vi "MENU_Shortcut Generate.vi"(6 "PlatMods":T3, 9 "VKey":T2, 10 "Char":i16) -> (2 "short cut":T1)   [LabVIEW 2016]
uses:
  <vilib>/event_ctls.llb/eventvkey.ctl
  <vilib>/Utility/miscctls.llb/LVMenuShortCut.ctl
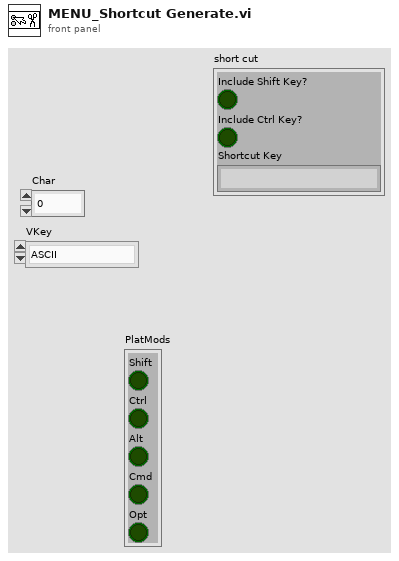
[diagram p1: front panel]
types:
  T1 = typedef "LVMenuShortCut.ctl" = cluster{"Include Shift Key?":bool, "Include Ctrl Key?":bool, "Shortcut Key":string}
  T2 = typedef "eventvkey.ctl" = enum16{"ASCII", "Enter", "Return", "Shift", "Ctrl", "Alt", "Cmd", "Opt", "Caps", "NumLock", "Clear", "Break", "Up", "Down", "Left", "Right", "Insert", "Delete", "Home", "End", "PageUp", "PageDown", "Escape", "Help", "Pause", "ScrollLock", "F1", "F2", "F3", "F4", "F5", "F6", "F7", "F8", "F9", "F10", "F11", "F12", "F13", "F14", "F15", "F16", "F17", "F18", "F19", "F20", "F21", "F22", "F23", "F24", "Play", "VolumeUp", "VolumeDown", "Mute", "Two Byte Char"}
  T3 = cluster{"Shift":bool, "Ctrl":bool, "Alt":bool, "Cmd":bool, "Opt":bool}
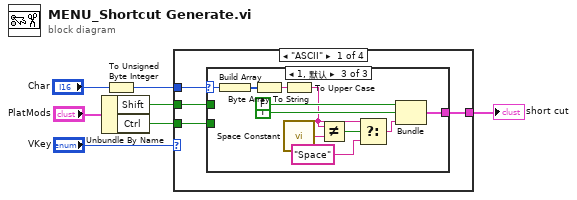
[diagram p0: block diagram]
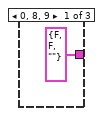
[diagram p2: hidden frame]
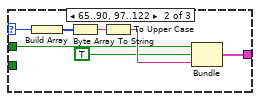
[diagram p3: hidden frame]
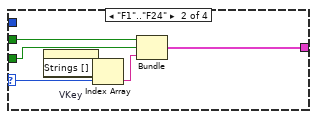
[diagram p4: hidden frame]
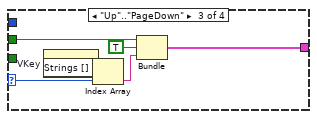
[diagram p5: hidden frame]
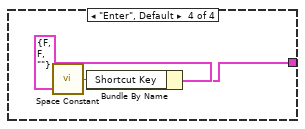
[diagram p6: hidden frame]
diagram:
  n1 = Unbundle By Name("PlatMods") -> ("Shift"=w4:bool, "Ctrl"=w3:bool)
  n2 = To Unsigned Byte Integer(number="Char") -> (unsigned 8bit integer=w2:u8)
  n3 = case shown="\"ASCII\"" "VKey" {
    selector: "VKey" -> [_ w35 w41 _]
    tunnel: w2 -> [w11 _ _ _]
    tunnel: w4 -> [w8 w34 w40 _]
    tunnel: w3 -> [w10 w33 _ _]
    tunnel: [w9 w31 w38 w43] -> w1
    frame "ASCII" {
      n4 = case shown="1, 默认" w11 {
        selector: w11 -> [_ w17 w28]
        tunnel: w10 -> [_ _ _]
        tunnel: [cluster{"Ctrl":bool, "Ctrl":bool, string} {"Ctrl"=FALSE, "Ctrl"=FALSE, ""} w16 w26] -> w9
        tunnel: w8 -> [_ w14 _]
        frame 0, 8, 9 {
        }
        frame 65..90, 97..122 {
          n5 = Build Array(w17) -> (w19:u8[])
          n6 = Byte Array To String(unsigned byte array=w19) -> (string=w18:string)
          n7 = To Upper Case(1:w18) -> (0:w15:string)
          n8 = Bundle("Shift"=w14, "Shift"=TRUE, w15) -> (w16:cluster{"Shift":bool, "Shift":bool, string})  [unwired: 1 in]
        }
        frame 1, Default {
          n9 = Build Array(w28) -> (w30:u8[])
          n10 = Byte Array To String(unsigned byte array=w30) -> (string=w29:string)
          n11 = To Upper Case(1:w29) -> (0:w22:string)
          n12 = call <vilib>:"Space Constant.vi"() -> ("String"=w24:string)
          n13 = Not Equal?(x=w22, y=w24) -> (x != y?=w23:bool)
          n14 = Select(t=w22, s=w23, f="Space") -> (s? t:f=w20:string)
          n15 = Bundle("Ctrl"=FALSE, "Shift"=TRUE, "f"=w20) -> (w26:cluster{"Ctrl":bool, "Shift":bool, "f":string})  [unwired: 1 in]
        }
      }
    }
    frame "F1".."F24" {
      n16 = property on="VKey" class="Enum (严格)"() -> ("Strings []"=w36:string[])  [unwired: 2 in, 2 out]
      n17 = Index Array(array=w36, index=w35) -> (element=w32:string)
      n18 = Bundle("Shift"=w34, "Ctrl"=w33, w32) -> (w31:cluster{"Shift":bool, "Ctrl":bool, string})  [unwired: 1 in]
    }
    frame "Up".."PageDown" {
      n19 = property on="VKey" class="Enum (严格)"() -> ("Strings []"=w42:string[])  [unwired: 2 in, 2 out]
      n20 = Index Array(array=w42, index=w41) -> (element=w39:string)
      n21 = Bundle("Shift"=w40, "Shift"=TRUE, w39) -> (w38:cluster{"Shift":bool, "Shift":bool, string})  [unwired: 1 in]
    }
    frame "Enter", Default {
      n22 = call <vilib>:"Space Constant.vi"() -> ("String"=w45:string)
      n23 = Bundle By Name(cluster=T1 {"Include Shift Key?"=FALSE, "Include Ctrl Key?"=FALSE, "Shortcut Key"=""} ("short cut"), "Shortcut Key"=w45) -> (w43:T1)
    }
  }
  "short cut" <- w1
